vi "random_array_element_single.vi"(1 "Array of numbers":sgl[](array[numeric]) format="%#_13g") -> (0 "Randomly selected number":sgl)   [LabVIEW 2019]
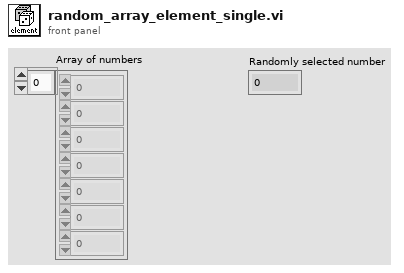
[diagram p1: front panel]
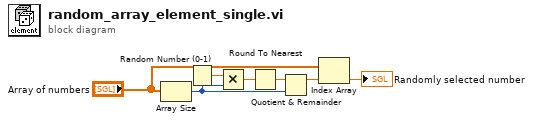
[diagram p0: block diagram]
diagram:
  n1 = Array Size(array="Array of numbers") -> (size(s)=w3:i32)
  n2 = Random Number (0-1)() -> (number: 0 to 1=w7:dbl)
  n3 = Multiply(x=w7, y=w3) -> (x*y=w6:dbl)
  n4 = Round To Nearest(number=w6) -> (nearest integer value=w5:dbl)
  n5 = Quotient & Remainder(x=w5, y=w3) -> (x-y*floor(x/y)=w4:dbl)  [unwired: 1 out]
  n6 = Index Array(array="Array of numbers", index=w4) -> (element=→"Randomly selected number":sgl)
